vi "Down-Right Vector Check.vi"(8 "Column":i32, 9 "Row":i32, 10 "Opponent's Tiles":bool[][](array[boolean]), 11 "Current Player's Tiles":bool[][](array[boolean])) -> (2 "Possible Flips":T1[](array[typedef]), 3 "Possible Location":bool)   [LabVIEW 2020, in "Reversi.lvlib" / "Reversi.lvclass"]
uses:
  Reversi.lvclass
  Space Coordinates.ctl
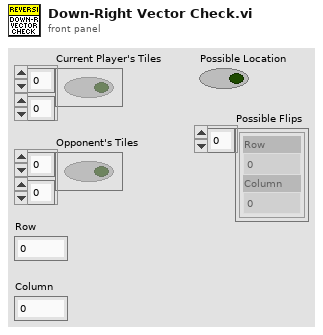
[diagram p1: front panel]
types:
  T1 = typedef "Reversi.lvlib/Reversi.lvclass/Space Coordinates.ctl" = cluster{"Row":i32, "Column":i32}
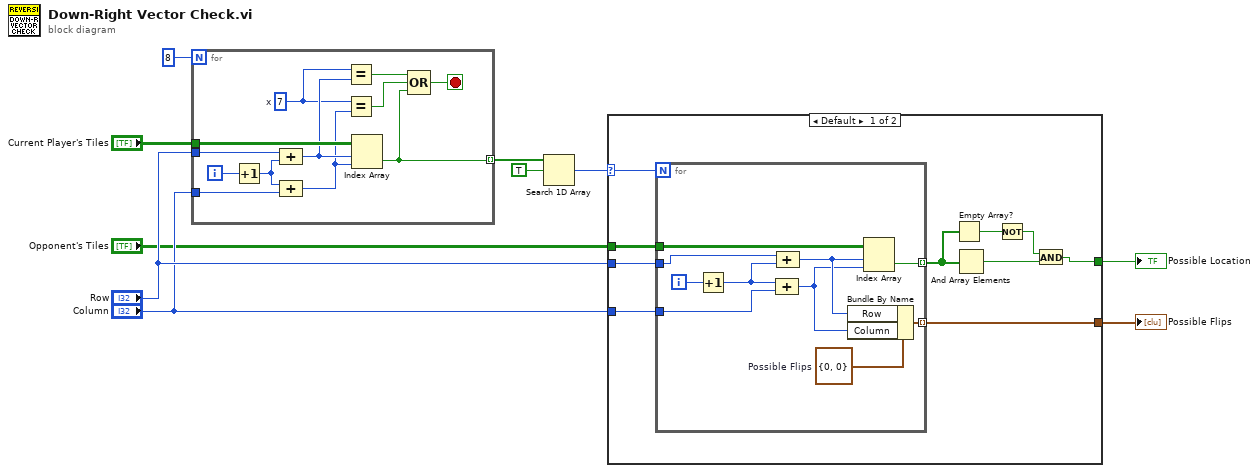
[diagram p0: block diagram]
diagram:
  n1 = for {
    N: 8 -> [_]
    tunnel: [w18] -> w9 mode=indexing
    tunnel: "Current Player's Tiles" -> [w22]
    tunnel: "Column" -> [w13]
    tunnel: "Row" -> [w20]
    i -> [w21]
    stop <- w17 stop-if-true
    w11 = 7  # x
    n2 = Increment(x=w21) -> (x+1=w14:i32)
    n3 = Compound Arithmetic op=ADD(w20, w14) -> (w15:i32)
    n4 = Compound Arithmetic op=ADD(w14, w13) -> (w12:i32)
    n5 = Equal?(x=w11, y=w15) -> (x = y?=w19:bool)
    n6 = Equal?(x=w11, y=w12) -> (x = y?=w16:bool)
    n7 = Index Array(array=w22, index (row)=w15, index (col)=w12) -> (element=w18:bool)
    n8 = Compound Arithmetic op=OR(w19, w16, w18) -> (w17:bool)
  }
  n9 = Search 1D Array(1D array=w9, element=TRUE) -> (index of element=w2:i32)  [unwired: 1 in]
  n10 = case shown="Default" w2 {
    selector: w2 -> [w23 _]
    tunnel: "Opponent's Tiles" -> [w28 _]
    tunnel: "Column" -> [w26 _]
    tunnel: [w29 _] -> w6
    tunnel: "Row" -> [w27 _]
    tunnel: [w24 _] -> w10
    frame Default {
      n11 = for {
        N: w23 -> [_]
        tunnel: [w40] -> w25 mode=indexing
        tunnel: w28 -> [w42]
        tunnel: w27 -> [w39]
        tunnel: w26 -> [w33]
        tunnel: [w38] -> w24 mode=indexing
        i -> [w41]
        w36 = T1 {"Row"=0, "Column"=0}  # Possible Flips
        n12 = Increment(x=w41) -> (x+1=w35:i32)
        n13 = Compound Arithmetic op=ADD(w35, w33) -> (w34:i32)
        n14 = Compound Arithmetic op=ADD(w39, w35) -> (w37:i32)
        n15 = Bundle By Name(cluster=w36, "Row"=w37, "Column"=w34) -> (w38:T1)
        n16 = Index Array(array=w42, index (row)=w37, index (col)=w34) -> (element=w40:bool)
      }
      n17 = Empty Array?(array=w25) -> (empty?=w32:bool)
      n18 = And Array Elements(Boolean array=w25) -> (logical AND=w30:bool)
      n19 = Not(x=w32) -> (.not. x?=w31:bool)
      n20 = And(x=w31, y=w30) -> (x .and. y?=w29:bool)
    }
    frame -1 {
    }
  }
  "Possible Flips" <- w10
  "Possible Location" <- w6
